vi "Query FFT Measurement Status.vi"(6 "Target Sync State (Adjusted)":i32(ring)=1 items=["Pending", "Adjusted"], 7 "Target Main State (Run)":i32(ring)=1 items=["Off", "Run", "Ready"], 8 "error in (no error)":errorcluster, 9 "Timeout (1)":i32=1 format="%.0g", 10 "Instance (1)":i32=1 format="%.0g", 11 "VISA resource name":refnum<visa-resource-name>) -> (0 "error out":errorcluster, 1 "Sync State":i32, 2 "Main State":i32, 3 "VISA resource name out":refnum<visa-resource-name>, 4 "Resources State":i32)   [LabVIEW 2020, in "Rohde&Schwarz CMXP GPRF.lvlib"]
doc: "Queries the main measurement state and the measurement substates.\n\nWithout query parameters, the states are returned immediately.\n\nWith query parameters, the states are returned when the <TargetMainState> and the <TargetSyncState> are reached or when the <Timeout> expires.\n\nAttribute:\nRSCMXPGPRF_ATTR_FFT_MEASUREMENT_STATUS_ALL\n\nRemote-control command:\nFETCh:GPRF:MEAS<i>:FFTSanalyzer:STATe:ALL?"
uses:
  <instrlib>/Rohde&Schwarz CMXP GPRF/Rohde&Schwarz CMXP GPRF.lvlib
  <instrlib>/Rohde&Schwarz CMXP GPRF/Private/rsidr_core.llb/rsidr_core.lvlib
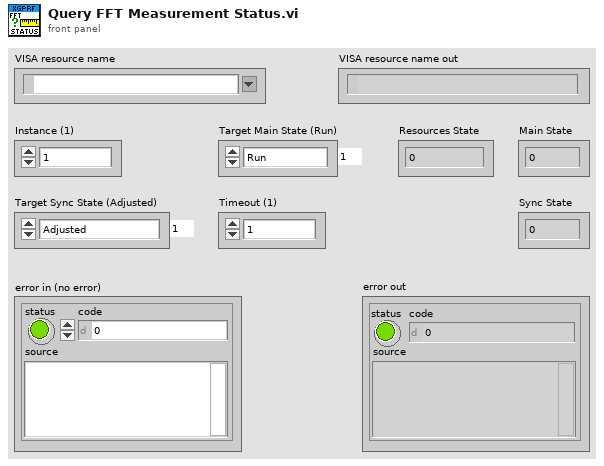
[diagram p1: front panel]
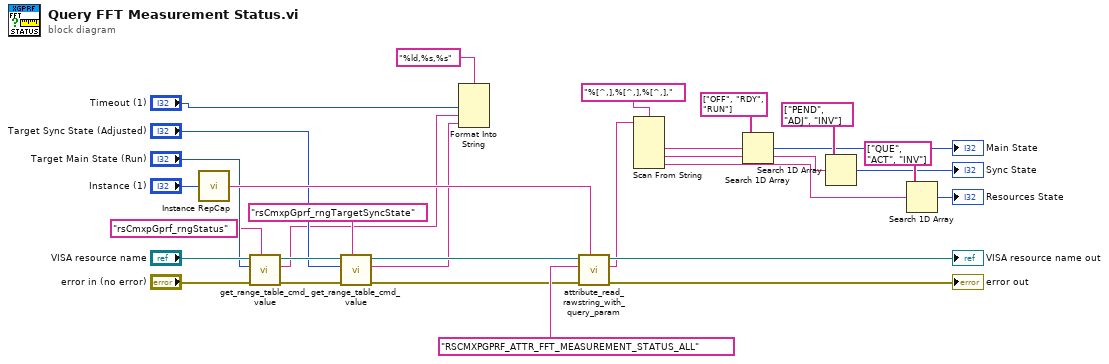
[diagram p0: block diagram]
diagram:
  n1 = call <instrlib>:"Instance RepCap.vi"("Instance in"="Instance (1)") -> ("Instance out"=w16:string)
  n2 = call <instrlib>:"get_range_table_cmd_value.vi"("Range Table ID in"="rsCmxpGprf_rngStatus", "error in"="error in (no error)", "Input Int32 value"="Target Main State (Run)", "VISA resource name"="VISA resource name") -> ("error out"=w12:errorcluster, "Cmd value out"=w2:string, "VISA resource name out"=w11:refnum<visa-resource-name>)  [unwired: 5 in]
  n3 = call <instrlib>:"get_range_table_cmd_value.vi"("Range Table ID in"="rsCmxpGprf_rngTargetSyncState", "error in"=w12, "Input Int32 value"="Target Sync State (Adjusted)", "VISA resource name"=w11) -> ("error out"=w10:errorcluster, "Cmd value out"=w1:string, "VISA resource name out"=w9:refnum<visa-resource-name>)  [unwired: 5 in]
  n4 = Format Into String(format string="%ld,%s,%s", "Timeout (1)", w2, w1) -> ()  [unwired: 2 in, 2 out]
  n5 = call <instrlib>:"attribute_read_rawstring_with_query_param.vi"("Repeated Capability (\"\")"=w16, "error in"=w10, "Attribute ID"="RSCMXPGPRF_ATTR_FFT_MEASUREMENT_STATUS_ALL", "VISA resource name"=w9) -> ("error out"=→"error out":errorcluster, "RawString out"=w15:string, "VISA resource name out"=→"VISA resource name out":refnum<visa-resource-name>)  [unwired: 5 in]
  n6 = Scan From String(format string="%[^,],%[^,],%[^,],", input string=w15) -> (output 1=w29:string, output 2=w21:string, output 3=w20:string)  [unwired: 5 in, 3 out]
  n7 = Search 1D Array(1D array=string[] ["OFF", "RDY", "RUN"], element=w29) -> (index of element=→"Main State":i32)  [unwired: 1 in]
  n8 = Search 1D Array(1D array=string[] ["PEND", "ADJ", "INV"], element=w21) -> (index of element=→"Sync State":i32)  [unwired: 1 in]
  n9 = Search 1D Array(1D array=string[] ["QUE", "ACT", "INV"], element=w20) -> (index of element=→"Resources State":i32)  [unwired: 1 in]
